vi "set_json_params.vi"(8 "error in (no error)":errorcluster caption="entrée d'erreur (pas d'erreur)", 10 "params":string, 11 "Model en entrée":refnum<class "Model.lvclass">) -> (0 "error out":errorcluster caption="sortie d'erreur", 3 "Model en sortie":refnum<class "Model.lvclass">)   [LabVIEW 2020, in "Model.lvclass"]
uses:
  Model.lvclass
  C:/Users/cipop/TDF Dropbox/2_Technologies de France/1 - Services et Etudes/PLAIY/2 - DEV/PLAIYLAB/code/Python/Python.lvclass
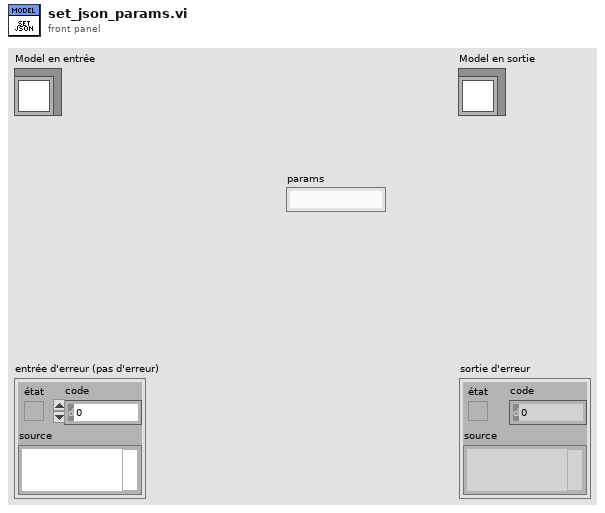
[diagram p1: front panel]
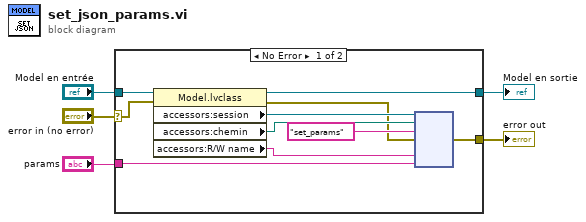
[diagram p0: block diagram]
diagram:
  n1 = case shown="No Error" "error in (no error)" {
    selector: "error in (no error)" -> [w12 w17]
    tunnel: [w14 w17] -> w4
    tunnel: [w6 w16] -> w2
    tunnel: "Model en entrée" -> [w13 w16]
    tunnel: "params" -> [w8 _]
    frame No Error {
      n2 = property class="Model.lvclass"(reference=w13, error in=w12) -> (reference out=w6:refnum<class "Model.lvclass">, error out=w7:errorcluster, "accessors:session"=w11:refnum<k35>, "accessors:chemin"=w10:path, "accessors:R/W name"=w9:string)
      n3 = node(w11, w10, "set_params" ("nom de la fonction"), w7, w9, w8) -> (w14:errorcluster)  [unwired: 4 in, 3 out]
    }
    frame Error {
    }
  }
  "error out" <- w4
  "Model en sortie" <- w2
